vi "Reorder String Array Breadth-firstly.vi"(11 "Array 3":string[](array[string])) -> (2 "Indexs":i32[](array[numeric]), 3 "Array":string[](array[string]))   [LabVIEW 2017, in "API String Arguments Support.lvlib"]
uses:
  API String Arguments Support.lvlib
  <userlib>/_NEVSTOP/Communicable State Machine(CSM)/Communicable State Machine.lvlib
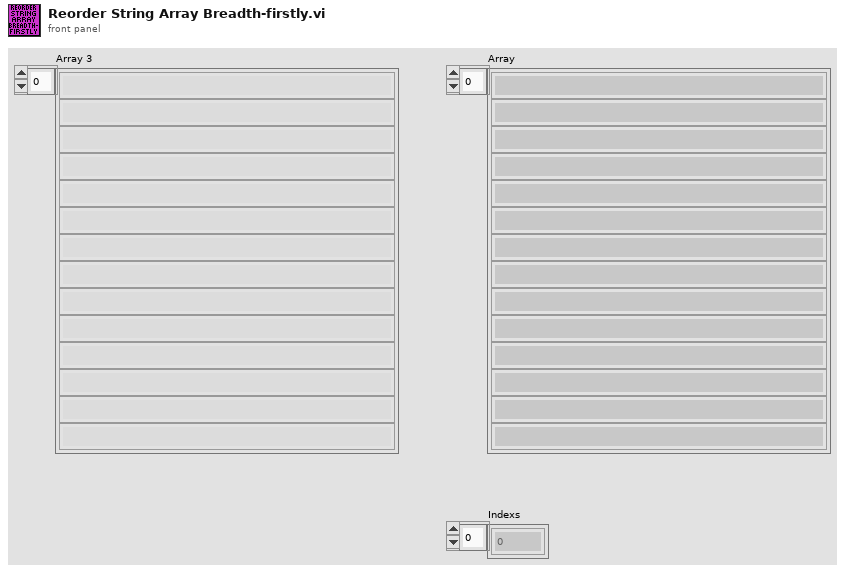
[diagram p1: front panel]
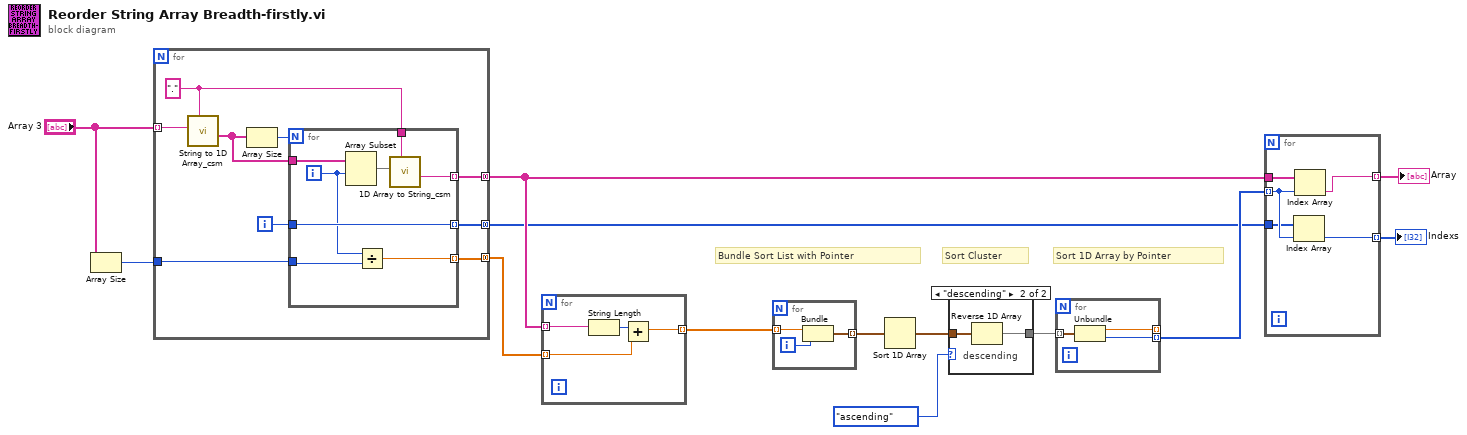
[diagram p0: block diagram]
diagram:
  # "Sort 1D Array by Pointer"
  # "Sort Cluster"
  # "Bundle Sort List with Pointer"
  n1 = Array Size(array="Array 3") -> (size(s)=w2:i32)
  n2 = for {
    tunnel: "Array 3" -> [w22] mode=indexing
    tunnel: [w19] -> w7 mode=concatenating
    tunnel: [w16] -> w4 mode=concatenating
    tunnel: w2 -> [w15]
    tunnel: [w14] -> w1 mode=concatenating
    i -> [w17]
    w18 = "." ("delimiter (Tab)")
    n3 = call <userlib>:"String to 1D Array_csm.vi"("delimiter (Tab)"=w18, "string"=w22) -> ("Array of Strings"=w20:string[])  [unwired: 9 in]
    n4 = Array Size(array=w20) -> (size(s)=w21:i32)
    n5 = for {
      N: w21 -> [_]
      tunnel: w20 -> [w30]
      tunnel: [w28] -> w19 mode=indexing
      tunnel: w18 -> [w27]
      tunnel: [w26] -> w16 mode=indexing
      tunnel: w17 -> [w26]
      tunnel: w15 -> [w25]
      tunnel: [w23] -> w14 mode=indexing
      i -> [w24]
      n6 = Array Subset(array=w30, index=w24) -> (w29:string[])  [unwired: 1 in]
      n7 = Divide(x=w24, y=w25) -> (x/y=w23:dbl)
      n8 = call <userlib>:"1D Array to String_csm.vi"("delimiter (Tab)"=w27, "Array of Strings"=w29) -> ("delimited string"=w28:string)  [unwired: 9 in]
    }
  }
  n9 = for {
    tunnel: w7 -> [w34] mode=indexing
    tunnel: [w33] -> w9 mode=indexing
    tunnel: w1 -> [w31] mode=indexing
    n10 = String Length(string=w34) -> (length=w32:i32)
    n11 = Add(x=w32, y=w31) -> (x+y=w33:dbl)
  }
  n12 = for {
    tunnel: w9 -> [w37] mode=indexing
    tunnel: [w35] -> w12 mode=indexing
    i -> [w36]
    n13 = Bundle(w37, w36) -> (w35:cluster{dbl, i32})  [unwired: 1 in]
  }
  n14 = Sort 1D Array(array=w12) -> (sorted array=w11:cluster{dbl, i32}[])
  n15 = case shown="\"descending\"" enum16{"ascending", "descending"}."ascending" ("Order") {
    tunnel: [w38 w39] -> w13
    tunnel: w11 -> [w38 w40]
    frame "ascending", Default {
    }
    frame "descending" {
      # "descending"
      n16 = Reverse 1D Array(array=w40) -> (reversed array=w39:cluster{dbl, i32}[])
    }
  }
  n17 = for {
    tunnel: w13 -> [w43] mode=indexing
    tunnel: [w41] -> _ mode=indexing
    tunnel: [w42] -> w10 mode=indexing
    n18 = Unbundle(w43) -> (w41:dbl, w42:i32)
  }
  n19 = for {
    tunnel: w7 -> [w48]
    tunnel: [w47] -> w8 mode=indexing
    tunnel: w10 -> [w46] mode=indexing
    tunnel: [w44] -> w5 mode=indexing
    tunnel: w4 -> [w45]
    n20 = Index Array(array=w45, index=w46) -> (element=w44:i32)
    n21 = Index Array(array=w48, index=w46) -> (element=w47:string)
  }
  "Array" <- w8
  "Indexs" <- w5
